vi "Custom Example.vi"() -> ()   [LabVIEW 2020]
uses:
  Source/Type Defs/Debug Level.ctl
  Custom Sink/Custom Sink.lvclass
  C:/Users/hughe_cx/Documents/05_repos/LVLog/Source/Sinks/Sink/Sink.lvclass
  Source/LV Log.lvlib
  Source/Logger/Logger.lvclass
panel:
  in  "error in (no error)":errorcluster
  in  "Debug Level":T1=enum."DEBUG"
  out "error out":errorcluster
  # "When creating a child of Sink, you can give your child Sink new parameters by  creating a constructor called New. See Custom Sink.vlclass for an example.\n\nOverride Log to implement specific logging Functionality. \n\nCustom Sink implements a 1 button dialog box as a demonstration"
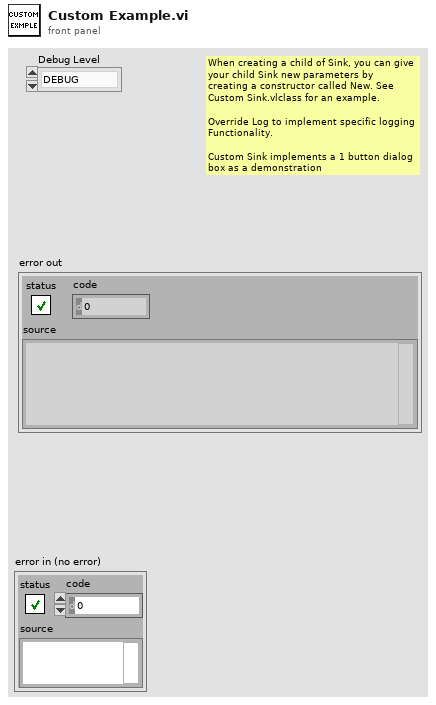
[diagram p1: front panel]
types:
  T1 = typedef "LV Log.lvlib/Debug Level.ctl" = enum16{"DEFAULT", "DEBUG", "INFO", "WARN", "ERROR", "FATAL"}
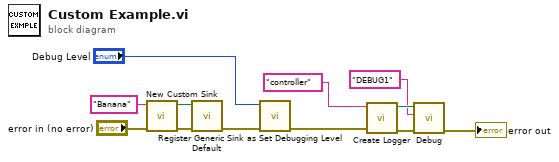
[diagram p0: block diagram]
diagram:
  n1 = call "New Custom Sink.vi"("error in (no error)"="error in (no error)", "Button Name"="Banana") -> ("error out"=w5:errorcluster, "Custom Sink out"=w6:refnum<class "Custom Sink.lvclass">)  [unwired: 8 in]
  n2 = call "Register Generic Sink as Default.vi"("error in (no error)"=w5, "Sink"=w6) -> ("error out"=w4:errorcluster)  [unwired: 9 in]
  n3 = call "Set Debugging Level.vi"("error in (no error)"=w4, "Debug Level in"="Debug Level") -> ("error out"=w10:errorcluster)  [unwired: 9 in]
  n4 = call "Create Logger.vi"("error in (no error)"=w10, "Name"="controller") -> ("error out"=w9:errorcluster, "Logger out"=w8:refnum<class "Logger.lvclass">)  [unwired: 8 in]
  n5 = call "Debug.vi"("error in (no error)"=w9, "Log Text"="DEBUG1", "Logger in"=w8) -> ("error out"=→"error out":errorcluster)  [unwired: 6 in, 2 out]
